vi "Read Data Packet.vi"(8 "error in (no error)":errorcluster, 11 "Control Box in":refnum<class "Control Box.lvclass">) -> (0 "error out":errorcluster, 1 "Bad Packet?":bool, 2 "Raw Data":u8[](array[numeric]), 3 "Control Box out":refnum<class "Control Box.lvclass">, 4 "Timeout?":bool)   [LabVIEW 2018, in "Control Box.lvlib" / "Control Box.lvclass"]
uses:
  Control Box.lvclass
  Control Box.lvclass/Control Box.ctl
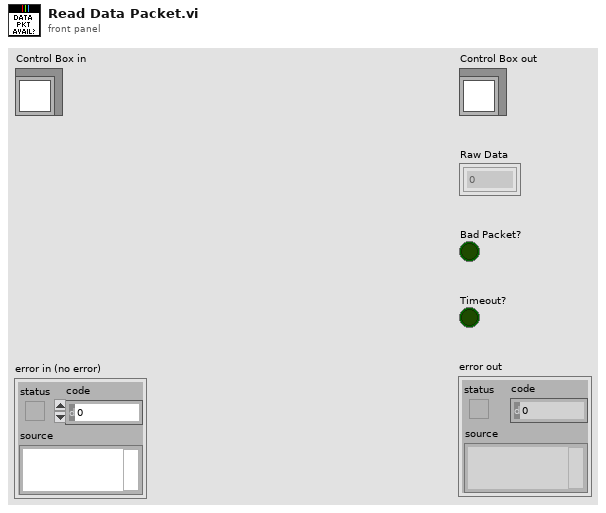
[diagram p1: front panel]
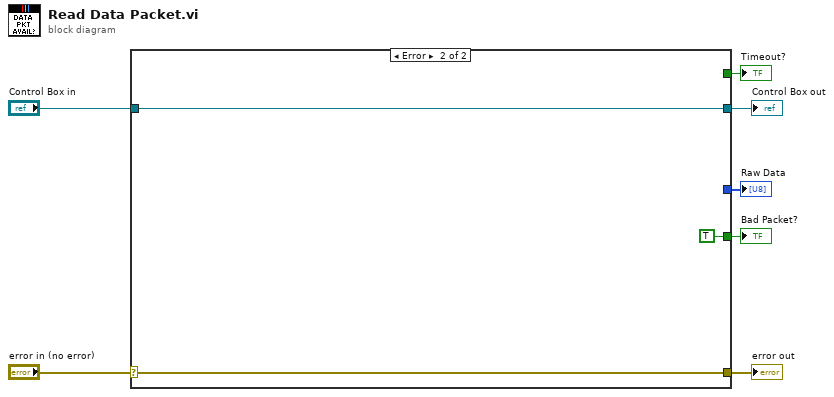
[diagram p0: block diagram]
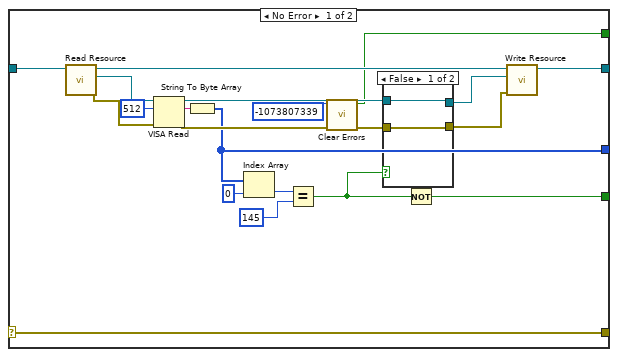
[diagram p2: hidden frame]
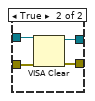
[diagram p3: hidden frame]
diagram:
  n1 = case shown="Error" "error in (no error)" {
    selector: "error in (no error)" -> [w28 w37]
    tunnel: [w28 w37] -> w6
    tunnel: [w25 w36] -> w4
    tunnel: "Control Box in" -> [w27 w36]
    tunnel: [w11 _] -> w3
    tunnel: [w10 _] -> w2
    tunnel: [w8 TRUE] -> w1
    frame No Error {
      n2 = call "Read Resource.vi"("Control Box in"=w27) -> ("error out"=w22:errorcluster, "Resource"=w24:refnum<visa-resource-name>, "Control Box out"=w26:refnum<class "Control Box.lvclass">)  [unwired: 8 in]
      n3 = VISA Read(VISA resource name=w24, byte count=u32 512, error in (no error)=w22) -> (VISA resource name out=w13:refnum<visa-resource-name>, read buffer=w21:string, error out=w20:errorcluster)  [unwired: 1 out]
      n4 = String To Byte Array(string=w21) -> (unsigned byte array=w11:u8[])
      n5 = Index Array(array=w11, index=0) -> (element=w17:u8)
      n6 = Equal?(x=w17, y=u8 145) -> (x = y?=w9:bool)
      n7 = call <vilib>:"Clear Errors.vi"("error in (no error)"=w20, "specific error code to clear (0: all)"=-1073807339) -> ("error out"=w15:errorcluster, "specific error cleared?"=w10:bool)  [unwired: 4 in]
      n8 = case shown="False" w9 {
        tunnel: w15 -> [w30 w34]
        tunnel: [w30 w33] -> w14
        tunnel: w13 -> [w29 w32]
        tunnel: [w29 w31] -> w12
        frame False {
        }
        frame True {
          n9 = VISA Clear(VISA resource name=w32, error in (no error)=w34) -> (VISA resource name out=w31:refnum<visa-resource-name>, error out=w33:errorcluster)
        }
      }
      n10 = Not(x=w9) -> (.not. x?=w8:bool)
      n11 = call "Write Resource.vi"("error in (no error)"=w14, "Resource"=w12, "Control Box in"=w26) -> ("Control Box out"=w25:refnum<class "Control Box.lvclass">)  [unwired: 7 in, 1 out]
    }
    frame Error {
    }
  }
  "error out" <- w6
  "Control Box out" <- w4
  "Raw Data" <- w3
  "Timeout?" <- w2
  "Bad Packet?" <- w1
